vi "Ejemplo6_Indicador_de_Alarmas.vi"() -> ()   [LabVIEW 2020]
panel:
  in  "Limite Min":dbl(slide) scale=0.0..100.0
  out "Aviso 3":string
  out "Aviso 2":string
  out "Alarma 3":bool
  out "Alarma 2":bool
  in  "Temp 3":u8(slide) scale=0.0..100.0
  in  "Temp 2":dbl(slide) scale=0.0..100.0
  out "Forma de Onda":dbl(graph)
  out "Aviso 1":string
  out "Alarma 1":bool
  in  "Limite Max":dbl(slide) scale=0.0..100.0
  in  "Temp 1":dbl(slide) scale=0.0..100.0
  # "Indicador de Alarmas"
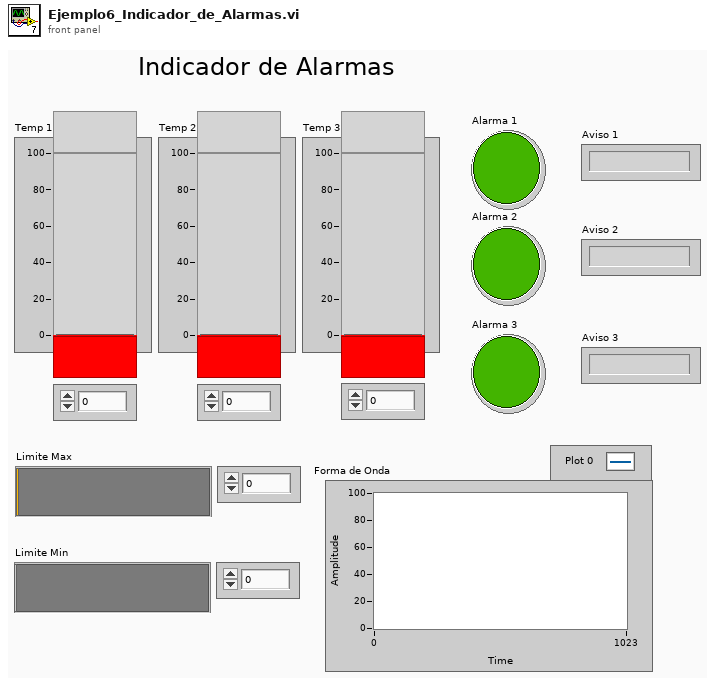
[diagram p1: front panel]
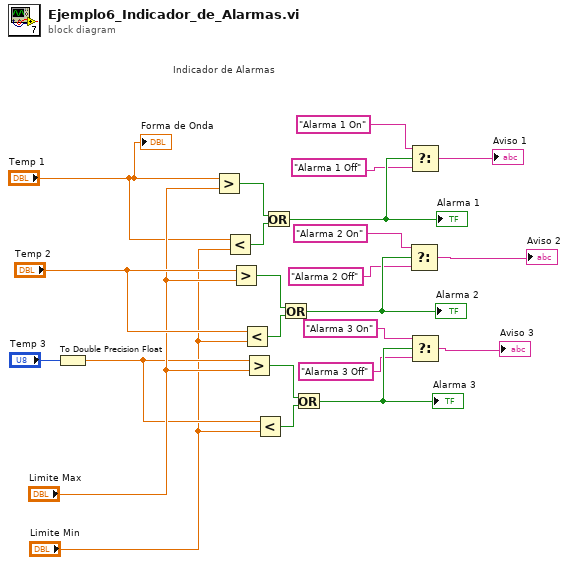
[diagram p0: block diagram]
diagram:
  # "Indicador de Alarmas"
  n1 = To Double Precision Float(number="Temp 3") -> (double precision float=w15:dbl)
  n2 = Greater?(x="Temp 1", y="Limite Max") -> (0:w24:bool)
  n3 = Less?(x="Temp 1", y="Limite Min") -> (x < y?=w23:bool)
  n4 = Greater?(x="Temp 2", y="Limite Max") -> (0:w22:bool)
  n5 = Less?(x="Temp 2", y="Limite Min") -> (x < y?=w21:bool)
  n6 = Greater?(x=w15, y="Limite Max") -> (0:w20:bool)
  n7 = Less?(x=w15, y="Limite Min") -> (x < y?=w19:bool)
  n8 = Or(x=w24, y=w23) -> (x .or. y?=w13:bool)
  "Alarma 1" <- w13
  n9 = Or(x=w22, y=w21) -> (x .or. y?=w12:bool)
  "Alarma 2" <- w12
  n10 = Or(x=w20, y=w19) -> (x .or. y?=w11:bool)
  "Alarma 3" <- w11
  n11 = Select(t="Alarma 2 On", s=w12, f="Alarma 2 Off") -> (s? t:f=→"Aviso 2":string)
  n12 = Select(t="Alarma 1 On", s=w13, f="Alarma 1 Off") -> (s? t:f=→"Aviso 1":string)
  n13 = Select(t="Alarma 3 On", s=w11, f="Alarma 3 Off") -> (s? t:f=→"Aviso 3":string)
  "Forma de Onda" <- "Temp 1"
